vi "VMUIStart.vi"(8 "error in (no error)":errorcluster, 10 "SubPanelRef":refnum<vi>, 11 "VariableManagerRef in":refnum<vi>) -> (0 "error out":errorcluster, 3 "VariableManagerRef out":refnum<vi>)   [LabVIEW 2013, in "VariableManagerAPI.lvlib"]
doc: "Start VariableManagerUserInterface. The user interface will be attached to the given sub panel reference.\n\nCreate a VariableManager object control in your application and give its referenct to this VI to start."
uses:
  VariableManagerAPI.lvlib
  VariableManager/VariableManager.lvclass
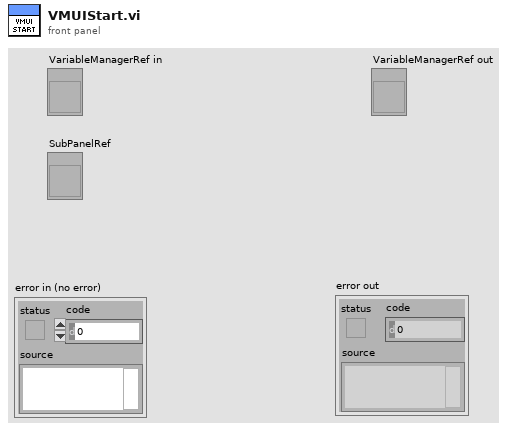
[diagram p1: front panel]
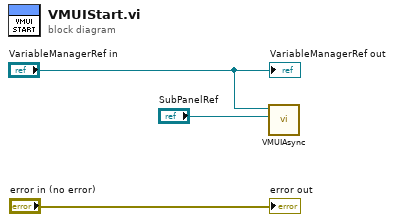
[diagram p0: block diagram]
diagram:
  n1 = call "VMUIAsync.vi"("SubPanelRef"="SubPanelRef", "VariableManagerRef in"="VariableManagerRef in") -> ()  [unwired: 10 in]
  "VariableManagerRef out" <- "VariableManagerRef in"
  "error out" <- "error in (no error)"
